vi "MonitorActiveProject.vi"(10 "Active Project Changed":refnum<user-event>) -> ()   [LabVIEW 2019]
doc: "Generates a user event when the active project in the current application instance changed. This VI keeps running until the specified user event is destroyed."
uses:
  b8ae5672-8134-400f-a408-93b2af799a79.vi
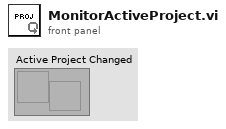
[diagram p1: front panel]
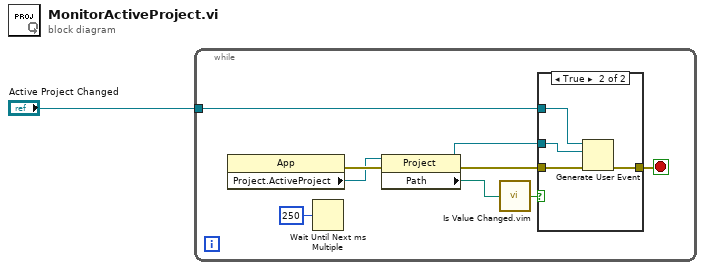
[diagram p0: block diagram]
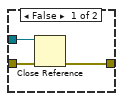
[diagram p2: hidden frame]
diagram:
  n1 = while {
    tunnel: "Active Project Changed" -> [w6]
    stop <- w3 stop-if-true
    n2 = property class="App"() -> (error out=w10:errorcluster, "Project.ActiveProject"=w9:refnum<vi>)  [unwired: 2 in, 1 out]
    n3 = Wait Until Next ms Multiple(millisecond multiple=u32 250) -> ()  [unwired: 1 out]
    n4 = property class="Project"(reference=w9, error in=w10) -> (reference out=w5:refnum<vi>, error out=w4:errorcluster, "Path"=w8:path)
    n5 = call "Is Value Changed.vim"("value"=w8) -> ("changed or first call?"=w7:bool)
    n6 = case shown="True" w7 {
      tunnel: w6 -> [_ w17]
      tunnel: w5 -> [w13 w16]
      tunnel: w4 -> [w12 w15]
      tunnel: [w11 w14] -> w3
      frame False {
        n7 = Close Reference(reference=w13, error in (no error)=w12) -> (error out=w11:errorcluster)
      }
      frame True {
        n8 = Generate User Event(user event=w17, event data cluster=w16, error in=w15) -> (error out=w14:errorcluster)  [unwired: 1 in, 1 out]
      }
    }
  }
